vi "Oriantation Update.vi"(1 "Oriantation Info In":T1) -> (0 "Oriantation Info Out":T1)   [LabVIEW 2013]
uses:
  Oritentation Global.vi
panel:
  # "The Horizontal \nVector of the \nCamera Mounts\nDistance"
  # "The Horizontal \nVector of the \nCamera Mounts\nDistance"
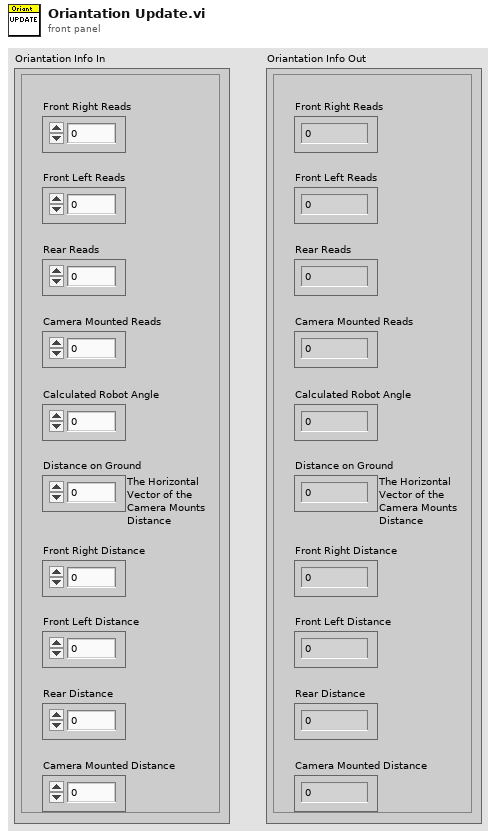
[diagram p1: front panel]
types:
  T1 = cluster{"Front Right Reads":dbl, "Front Left Reads ":dbl, "Rear Reads":dbl, "Camera Mounted Reads":dbl, "Calculated Robot Angle":dbl, "Distance on Ground":dbl, "Front Right Distance":dbl, "Front Left Distance":dbl, "Rear Distance":dbl, "Camera Mounted Distance":dbl}
  T2 = typedef "WPI_AnalogChannelDevRef.ctl" = cluster{"DevStatus":errorcluster, "Analog Module":T3, "Analog Channel":T4}
  T3 = typedef "FPGA_TypedefAnalogModule.ctl" = enum16{"Analog Module 1", "Analog Module 2"}
  T4 = typedef "FPGA_AIChannel.ctl" = enum8{"AI 1", "AI 2", "AI 3", "AI 4", "AI 5", "AI 6", "AI 7", "AI 8", "Invalid"}
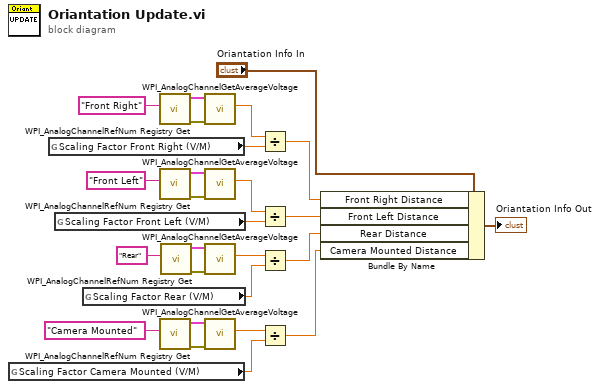
[diagram p0: block diagram]
diagram:
  n1 = global read "Oritentation Global.vi" "Scaling Factor Camera Mounted (V/M)"() -> (w13:dbl)
  n2 = global read "Oritentation Global.vi" "Scaling Factor Front Right (V/M)"() -> (w10:dbl)
  n3 = global read "Oritentation Global.vi" "Scaling Factor Front Left (V/M)"() -> (w9:dbl)
  n4 = global read "Oritentation Global.vi" "Scaling Factor Rear (V/M)"() -> (w11:dbl)
  n5 = call <vilib>:"WPI_AnalogChannelRefNum Registry Get.vi"("refnum name"="Front Right") -> ("error out"=w18:errorcluster, "AIDeviceRef"=w17:T2)  [unwired: 9 in]
  n6 = call <vilib>:"WPI_AnalogChannelRefNum Registry Get.vi"("refnum name"="Front Left") -> ("error out"=w16:errorcluster, "AIDeviceRef"=w15:T2)  [unwired: 9 in]
  n7 = call <vilib>:"WPI_AnalogChannelRefNum Registry Get.vi"("refnum name"="Camera Mounted") -> ("error out"=w22:errorcluster, "AIDeviceRef"=w21:T2)  [unwired: 9 in]
  n8 = call <vilib>:"WPI_AnalogChannelRefNum Registry Get.vi"("refnum name"="Rear") -> ("error out"=w20:errorcluster, "AIDeviceRef"=w19:T2)  [unwired: 9 in]
  n9 = call <vilib>:"WPI_AnalogChannelGetAverageVoltage.vi"("error in (no error)"=w18, "AIDeviceRef"=w17) -> ("Voltage"=w6:dbl)  [unwired: 9 out]
  n10 = call <vilib>:"WPI_AnalogChannelGetAverageVoltage.vi"("error in (no error)"=w16, "AIDeviceRef"=w15) -> ("Voltage"=w4:dbl)  [unwired: 9 out]
  n11 = call <vilib>:"WPI_AnalogChannelGetAverageVoltage.vi"("error in (no error)"=w20, "AIDeviceRef"=w19) -> ("Voltage"=w8:dbl)  [unwired: 9 out]
  n12 = call <vilib>:"WPI_AnalogChannelGetAverageVoltage.vi"("error in (no error)"=w22, "AIDeviceRef"=w21) -> ("Voltage"=w14:dbl)  [unwired: 9 out]
  n13 = Divide(x=w6, y=w10) -> (x/y=w5:dbl)
  n14 = Divide(x=w4, y=w9) -> (x/y=w3:dbl)
  n15 = Divide(x=w8, y=w11) -> (x/y=w7:dbl)
  n16 = Divide(x=w14, y=w13) -> (x/y=w12:dbl)
  n17 = Bundle By Name(cluster="Oriantation Info In", "Front Right Distance"=w5, "Front Left Distance"=w3, "Rear Distance"=w7, "Camera Mounted Distance"=w12) -> (→"Oriantation Info Out":T1)
